vi "writeFromeQueue.vi"(8 "queue":refnum<queue>, 11 "Cluster":T2) -> (0 "output cluster":T1, 3 "GCODE WAIT   2":i32)   [LabVIEW 2017]
uses:
  mWorkToolkit/libSerial/stateSerialUltra.ctl
panel:
  out "Data Write":string
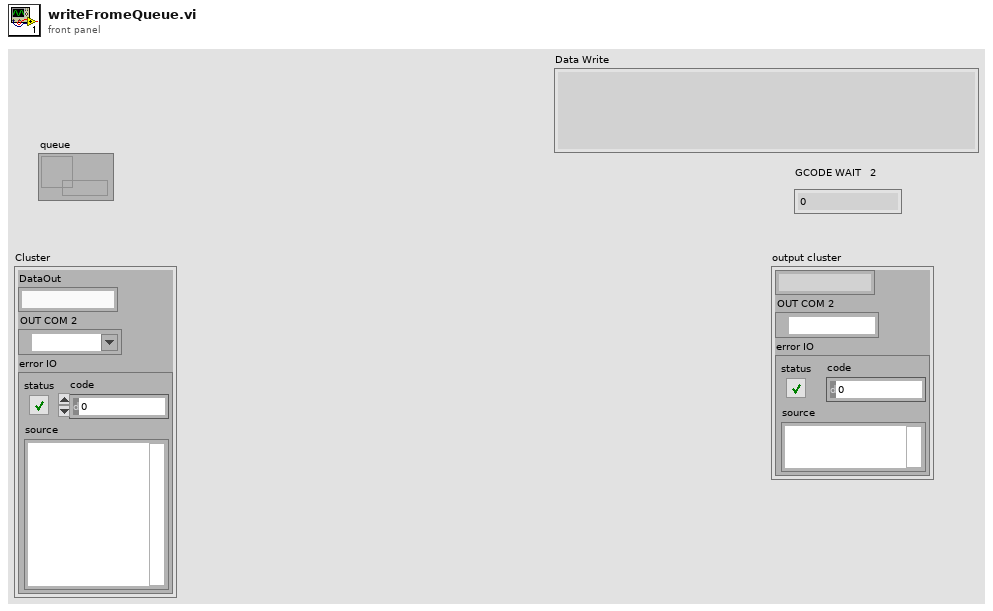
[diagram p1: front panel]
types:
  T1 = cluster{string, "OUT COM 2":refnum<visa-resource-name>, "error IO":errorcluster}
  T2 = cluster{"DataOut":string, "OUT COM 2":refnum<visa-resource-name>, "error IO":errorcluster}
  T3 = typedef "stateSerialUltra.ctl" = enum16{"findCOM", "Init", "CheckConnect", "Read", "Write", "exit"}
  T4 = cluster{string, "OUT COM 2":refnum<visa-resource-name>, "error out":errorcluster}
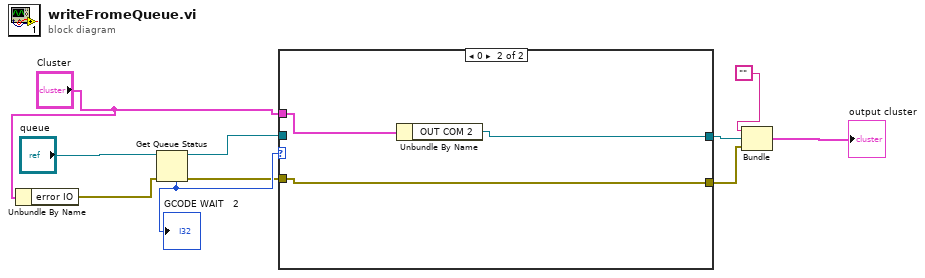
[diagram p0: block diagram]
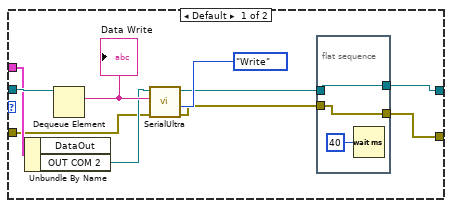
[diagram p2: hidden frame]
diagram:
  n1 = Unbundle By Name("Cluster") -> ("error IO"=w1:errorcluster)
  n2 = Get Queue Status(queue="queue", error in (no error)=w1) -> (queue out=w6:refnum<queue>, error out=w2:errorcluster, # elements in queue=w7:i32)  [unwired: 1 in, 5 out]
  "GCODE WAIT   2" <- w7
  n3 = case shown="0" w7 {
    tunnel: [w14 w24] -> w9
    tunnel: [w13 w25] -> w10
    tunnel: w6 -> [w18 _]
    tunnel: "Cluster" -> [w17 w26]
    tunnel: w2 -> [w11 w24]
    frame Default {
      n4 = Unbundle By Name(w17) -> ("OUT COM 2"=w16:refnum<visa-resource-name>)  [unwired: 1 out]
      n5 = Dequeue Element(queue=w18) -> (element=w20:string)  [unwired: 2 in, 3 out]
      "Data Write" <- w20
      n6 = call "SerialUltra.vi"("error in"=w11, "State"=stateSerialUltra."Write", "Data Write"=w20, "IN COM"=w16) -> ("error out"=w15:errorcluster, "OUT COM 2"=w12:refnum<visa-resource-name>)  [unwired: 3 in, 3 out]
      n7 = flat-sequence {
        tunnel: w15 -> [w23]
        tunnel: [w23] -> w14
        tunnel: [w21] -> w13
        tunnel: w12 -> [w21]
        frame #0 {
          n8 = Wait (ms)(milliseconds to wait=u32 40) -> ()  [unwired: 1 out]
        }
      }
    }
    frame 0 {
      n9 = Unbundle By Name(w26) -> ("OUT COM 2"=w25:refnum<visa-resource-name>)
    }
  }
  n10 = Bundle("", "OUT COM 2"=w10, "error out"=w9) -> (→"output cluster":T4)  [unwired: 1 in]
